vi "Set PMTs.vi"(8 "Error In":errorcluster, 10 "PMT 2":T1 max=1000 step=5 scale=0.0..1000.0, 11 "PMT 1":T1 max=1000 step=5 scale=0.0..1000.0) -> (0 "Error Out":errorcluster)   [LabVIEW 2013]
uses:
  Typedefs/PMT control knob.ctl
  Typedefs/HW config states enum.ctl
  <vilib>/DAQmx/write.llb/DAQmx Write (Analog 1D DBL NChan 1Samp).vi
  <vilib>/DAQmx/create/channels.llb/DAQmx Create Channel (AO-Voltage-Basic).vi
  <vilib>/DAQmx/miscellaneous.llb/DAQmx Fill In Error Info.vi
panel:
  out "DAQmx Physical Channel":tag="PXI1Slot4/ao2:3"
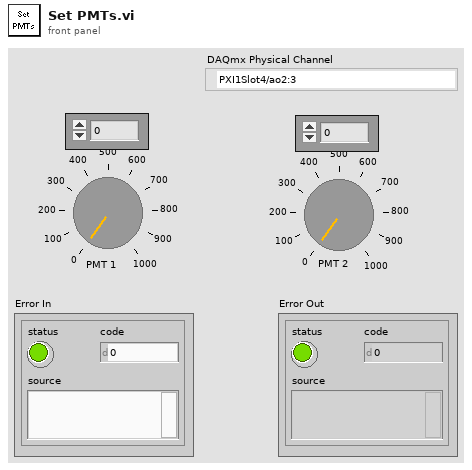
[diagram p1: front panel]
types:
  T1 = typedef "PMT control knob.ctl" = u16
  T2 = typedef "HW config states enum.ctl" = enum16{"Load from file", "Save to file", "Write all", "Read all", "Write XY stage settings", "Write DAQ FPGA settings", "Write Control FPGA settings", "Write Phys Channels", "Clear", "Compare from file"}
  T3 = typedef "Sys Configuration.ctl" = cluster{"XY Stage":T4, "DAQ FPGA":T5, "Control system":T9, "Encoder":T10, "DAQmx Chan":T11, "Computer MAC address":string, "Cam VidRec":T12, "Externalise Triggers":bool, "Laser wavelength (nm)":dbl}
  T4 = typedef "XY Stage config cluster.ctl" = cluster{"COM port":refnum<visa-resource-name>, "XY stage available":bool}
  T5 = typedef "DAQ FPGA config cluster.ctl" = cluster{"Ref":T6, "Target":T7, "Clock Freq (MHz) ":dbl, "input card type":T8, "Samples Wait after Trigger":u16, "AOD fill":u16, "StartupDelay":i32, "Slip Cycle (clock cycles)":u32, "Add Cycle":bool}
  T6 = typedef "FPGA Ref.ctl" = refnum<k20>
  T7 = typedef "nirio_resource_hc.ctl" = tag
  T8 = typedef "FPGA input type AC-DC.ctl" = enum16{"AC Card", "DC Card"}
  T9 = typedef "CTRL system config cluster.ctl" = cluster{"Ethernet opened":bool, "Ethernet Port":u32, "Ctrl FPGA available":bool, "Ctrl FPGA Clock (MHz)":dbl, "Ctrl system MAC address":string, "Control system.Network adapter name":string, "AOD 1 Amplitude":i16, "AOD 2 Amplitude":i16, "AOD 3 Amplitude":i16, "AOD 4 Amplitude":i16, "Data Time Interval (ns)":dbl, "T0 (ns)":dbl, "Ta (ns)":dbl}
  T10 = typedef "Encoder config cluster.ctl" = cluster{"IP address":string, "Port":u16, "Encoder available":bool, "Wheel radius (cm)":dbl}
  T11 = typedef "DAQmx physical channels cluster.ctl" = cluster{"Pockels AO":tag, "Hard shutter AO":tag, "PMT AOs":tag, "Power meter AI":tag}
  T12 = typedef "Cam VidRec HW config setup cluster.ctl" = cluster{"DO flag-Video record":tag, "DO flag-Trial start":tag, "VidRec available":bool}
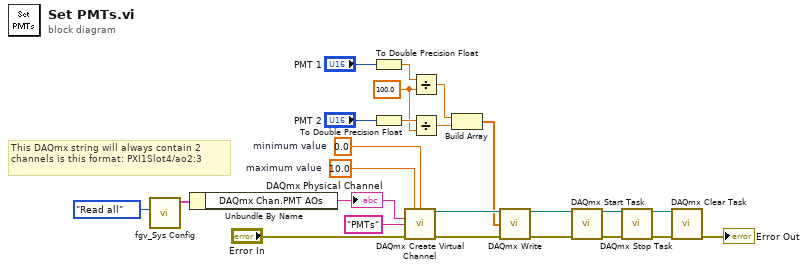
[diagram p0: block diagram]
diagram:
  w4 = 100.0 ("y")
  w15 = 10.0  # maximum value
  w16 = 0.0  # minimum value
  # "This DAQmx string will always contain 2 channels is this format: PXI1Slot4/ao2:3"
  n1 = call "fgv_Sys Config.vi"("Function"=HW_config_states_enum."Read all") -> ("System Config out"=w2:T3)  [unwired: 9 in, 1 out]
  n2 = Unbundle By Name(w2) -> ("DAQmx Chan.PMT AOs"=w1:tag)
  "DAQmx Physical Channel" <- w1
  n3 = To Double Precision Float(number="PMT 1") -> (double precision float=w5:dbl)
  n4 = To Double Precision Float(number="PMT 2") -> (double precision float=w6:dbl)
  n5 = call-poly <vilib>:"DAQmx Create Virtual Channel.vi"("maximum value"=w15, "minimum value"=w16, "physical channels"=w1, "name to assign"="PMTs", "error in"="Error In") -> ("task out"=w24:refnum<k21>, "error out"=w23:errorcluster)  [unwired: 9 in]
  n6 = Divide(x=w5, y=w4) -> (x/y=w11:dbl)
  n7 = Divide(x=w6, y=w4) -> (x/y=w8:dbl)
  n8 = Build Array(w11, w8) -> (w7:dbl[])
  n9 = call-poly <vilib>:"DAQmx Write.vi"("task/channels in"=w24, "data"=w7, "error in"=w23) -> ("task out"=w22:refnum<k21>, "error out"=w21:errorcluster)  [unwired: 10 in, 1 out]
  n10 = call <vilib>:"DAQmx Start Task.vi"("task/channels in"=w22, "error in"=w21) -> ("task out"=w13:refnum<k21>, "error out"=w14:errorcluster)  [unwired: 12 in]
  n11 = call <vilib>:"DAQmx Stop Task.vi"("task/channels in"=w13, "error in"=w14) -> ("task out"=w20:refnum<k21>, "error out"=w19:errorcluster)  [unwired: 12 in]
  n12 = call <vilib>:"DAQmx Clear Task.vi"("task in"=w20, "error in"=w19) -> ("error out"=→"Error Out":errorcluster)  [unwired: 13 in]
